vi "Render.vi"(8 "error in (no error)":errorcluster, 10 "String in":string, 11 "LinkingHeadingId in":refnum<class "LinkingHeadingId.lvclass">) -> (0 "error out":errorcluster, 2 "String out":string, 3 "LinkingHeadingId out":refnum<class "LinkingHeadingId.lvclass">)   [LabVIEW 2021, in "LvMarkdown.lvlib" / "LinkingHeadingId.lvclass"]
uses:
  LinkingHeadingId.lvclass
  LinkingHeadingId.lvclass/LinkingHeadingId.ctl
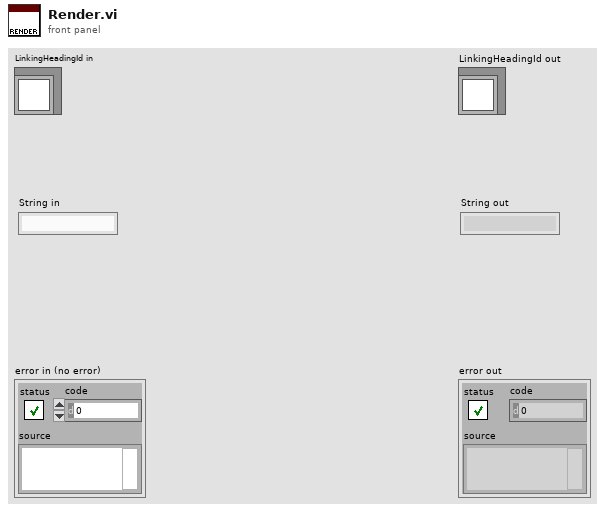
[diagram p1: front panel]
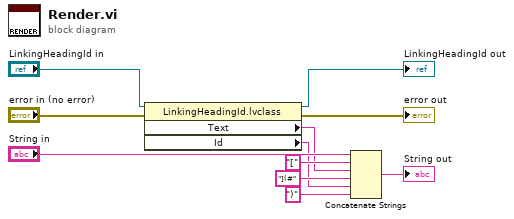
[diagram p0: block diagram]
diagram:
  n1 = property class="LinkingHeadingId.lvclass"(reference="LinkingHeadingId in", error in="error in (no error)") -> (reference out=→"LinkingHeadingId out":refnum<class "LinkingHeadingId.lvclass">, error out=→"error out":errorcluster, "Text"=w9:string, "Id"=w7:string)
  n2 = Concatenate Strings("String in", "[" ("string"), w9, "](#" ("string"), w7, ")" ("string")) -> (→"String out":string)
